vi "Get and Format debug data.vi"(7 "Table Control refnum":refnum<vi>, 9 "Update table position?":bool=TRUE, 10 "Format debug data?":bool, 11 "Empty debug data?":bool) -> (2 "Formatted debug data":string, 3 "Debug data array":T1[](array[typedef]) {"Time Stamp" format="%<%.3X %x>T"})   [LabVIEW 2019, in "ACSVcontrol-driver.lvlib"]
doc: "If debug mode was set on (use Initialize Globals), VI returns debug data.\nClears debug data if set.\nReturns debug data formatted as tab separated text if set.\nIf Table refnum exist, adds debug data into table. If set, the last shown row of the table is moved to show last row.\n\nDebug data are:\n- Time stamp\n- Write or Read\n- Status of Labview error after writing/reading all data\n- Data (TCP/IP message)\n- Code of Labview error\n- Source of Labview error\n- Call chain"
uses:
  ACSVcontrol-driver.lvlib
  Private/Type definitions/Debug data.ctl
  Private/Globals.vi
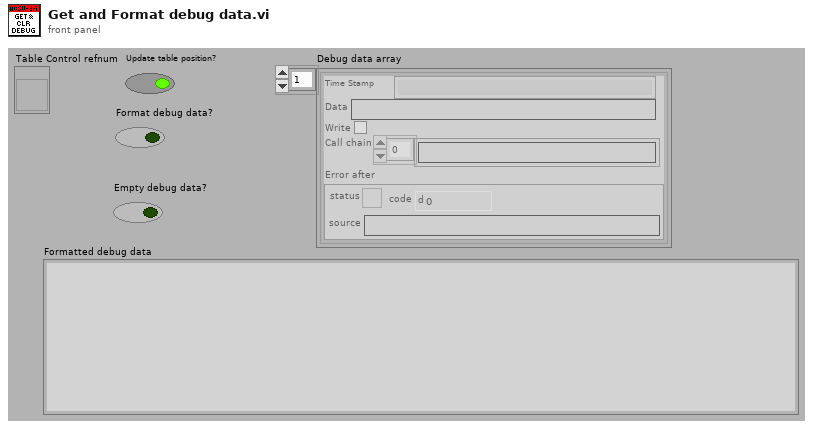
[diagram p1: front panel]
types:
  T1 = typedef "ACSVcontrol-driver.lvlib/Debug data.ctl" = cluster{"Time Stamp":timestamp, "Data":string, "Write":bool, "Call chain":string[], "Error after":errorcluster}
  T2 = typedef "LVRowAndColumnUnsignedTypeDef.ctl" = cluster{"Row":u32, "Column":u32}
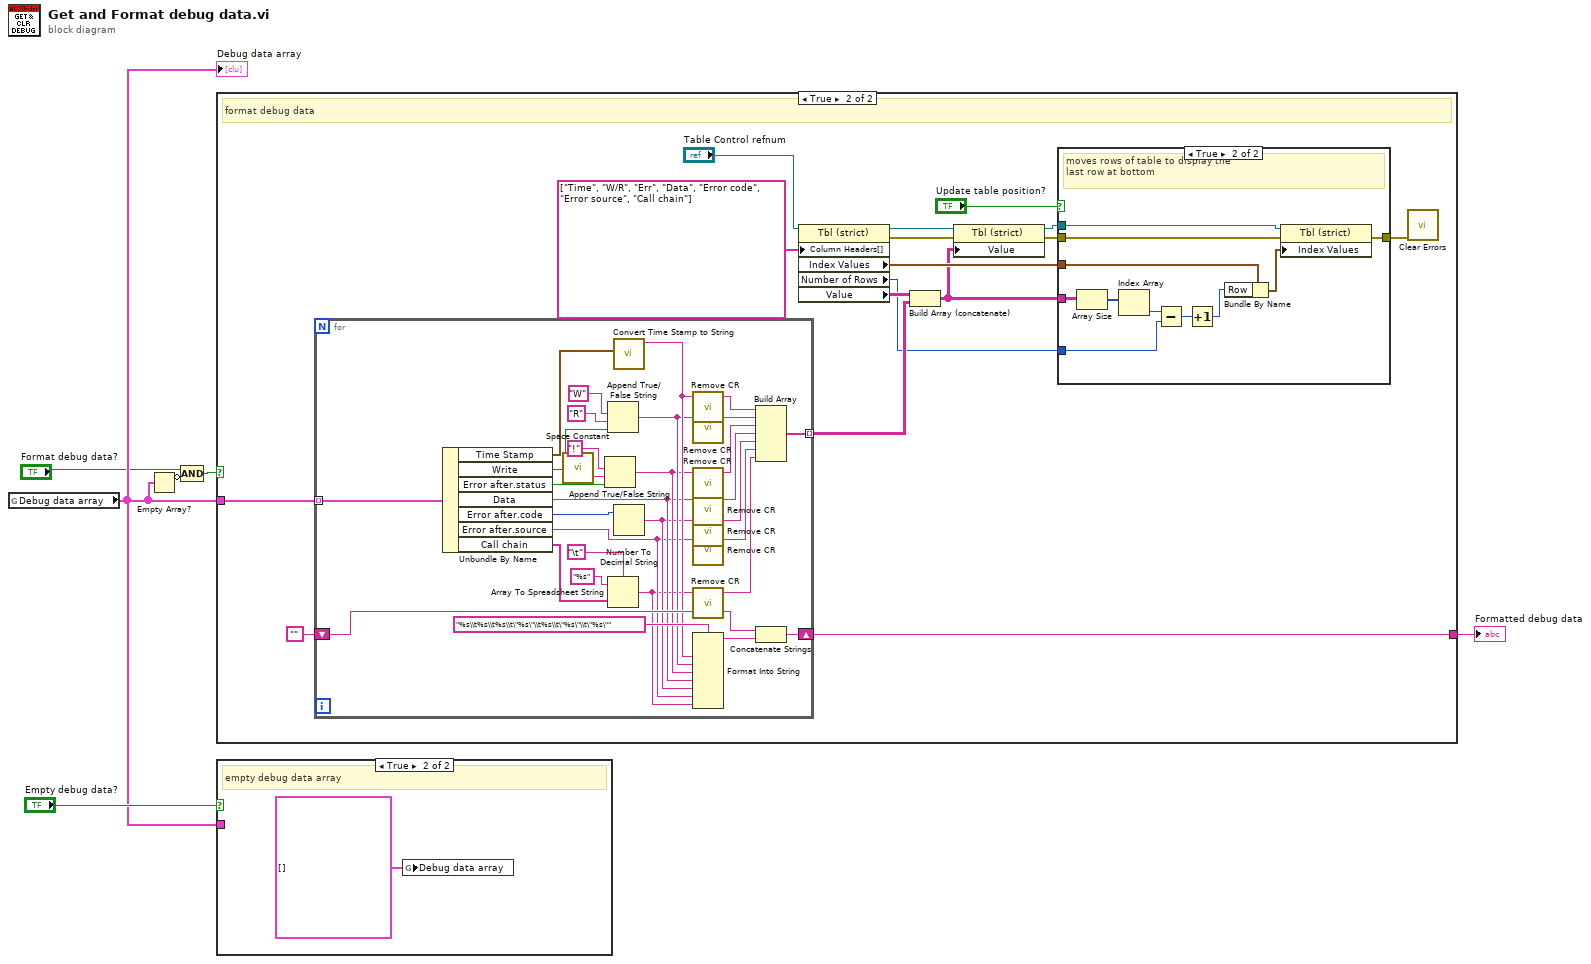
[diagram p0: block diagram]
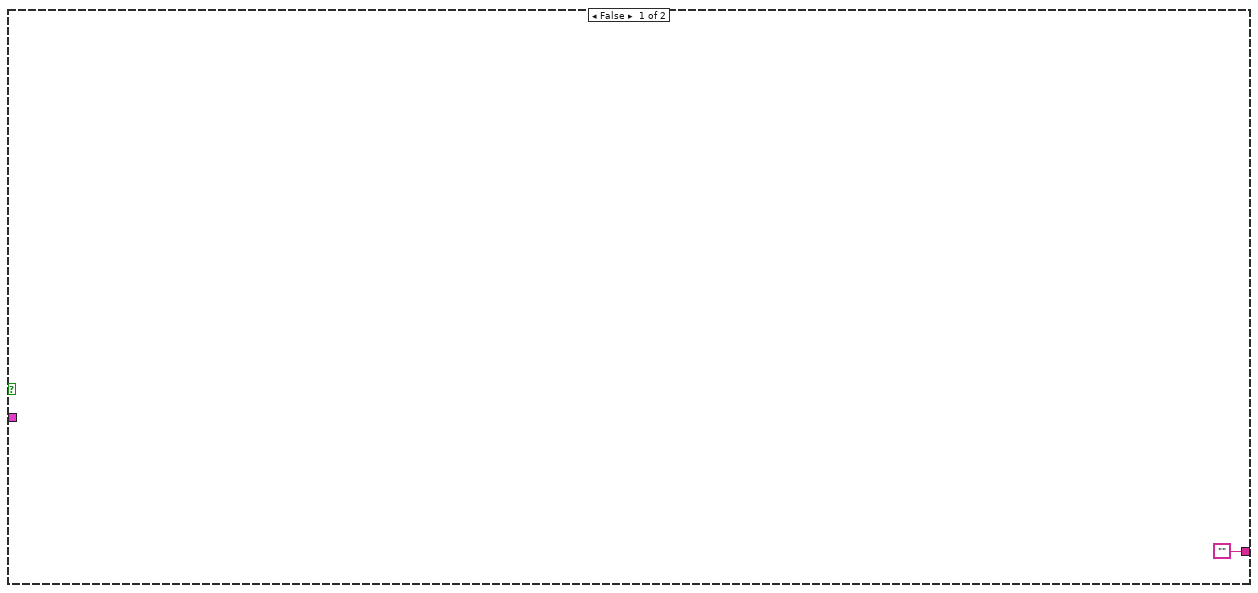
[diagram p2: hidden frame]
diagram:
  n1 = global read "Globals.vi" "Debug data array"() -> (w4:T1[])
  "Debug data array" <- w4
  n2 = Empty Array?(array=w4) -> (empty?=w3:bool)
  n3 = Compound Arithmetic op=AND("Format debug data?", invert w3) -> (w1:bool)
  n4 = case shown="True" w1 {
    tunnel: w4 -> [_ w23]
    tunnel: ["" w21] -> w5
    frame False {
    }
    frame True {
      # "format debug data"
      n5 = for {
        tunnel: w23 -> [w66] mode=indexing
        shift-right: [w54] -> w21
        shift-left: "" -> [w55]
        tunnel: [w53] -> w20 mode=indexing
        n6 = Unbundle By Name(w66) -> ("Time Stamp"=w65:timestamp, "Write"=w61:bool, "Error after.status"=w50:bool, "Data"=w46:string, "Error after.code"=w51:i32, "Error after.source"=w44:string, "Call chain"=w52:string[])
        n7 = call <vilib>:"Space Constant.vi"() -> ("String"=w59:string)
        n8 = Append True/False String(1:w50, 2:w59, 3:"!" ("true string")) -> (0:w47:string)  [unwired: 1 in]
        n9 = Append True/False String(1:w61, 2:"R" ("false string"), 3:"W" ("true string")) -> (0:w48:string)  [unwired: 1 in]
        n10 = Array To Spreadsheet String(delimiter (Tab)="\t", array=w52, 3:"%s" ("format string")) -> (spreadsheet string=w43:string)
        n11 = call "Convert Time Stamp to String.vi"("time stamp"=w65) -> ("date/time string"=w49:string)  [unwired: 10 in]
        n12 = Number To Decimal String(number=w51) -> (decimal integer string=w45:string)  [unwired: 1 in]
        n13 = call "Remove CR.vi"("string"=w49) -> ("string out"=w36:string)  [unwired: 4 in]
        n14 = call "Remove CR.vi"("string"=w48) -> ("string out"=w37:string)  [unwired: 4 in]
        n15 = call "Remove CR.vi"("string"=w47) -> ("string out"=w38:string)  [unwired: 4 in]
        n16 = call "Remove CR.vi"("string"=w46) -> ("string out"=w39:string)  [unwired: 4 in]
        n17 = call "Remove CR.vi"("string"=w45) -> ("string out"=w40:string)  [unwired: 4 in]
        n18 = call "Remove CR.vi"("string"=w44) -> ("string out"=w41:string)  [unwired: 4 in]
        n19 = call "Remove CR.vi"("string"=w43) -> ("string out"=w42:string)  [unwired: 4 in]
        n20 = Format Into String(format string="%s\\t%s\\t%s\\t\"%s\"\\t%s\\t\"%s\"\\t\"%s\"", w49, w48, w47, w46, w45, w44, w43) -> (resulting string=w56:string)  [unwired: 2 in, 1 out]
        n21 = Build Array(w36, w37, w38, w39, w40, w41, w42) -> (w53:string[])
        n22 = Concatenate Strings(w55, w56) -> (w54:string)
      }
      n23 = property class="Tbl (strict)"(reference="Table Control refnum", "Column Headers[]"=string[] ["Time", "W/R", "Err", "Data", "Error code", "Error source", "Call chain"] ("appended array")) -> (reference out=w16:refnum<vi>, error out=w15:errorcluster, "Index Values"=w18:T2, "Number of Rows"=w13:u32, "Value"=w19:string[][])  [unwired: 1 in]
      n24 = Build Array (concatenate)(w19, w20) -> (w12:string[][])
      n25 = property class="Tbl (strict)"(reference=w16, error in=w15, "Value"=w12) -> (reference out=w17:refnum<vi>, error out=w14:errorcluster)
      n26 = case shown="True" "Update table position?" {
        tunnel: w18 -> [_ w35]
        tunnel: w17 -> [_ w33]
        tunnel: w14 -> [w24 w32]
        tunnel: w13 -> [_ w31]
        tunnel: w12 -> [_ w30]
        tunnel: [w24 w25] -> w9
        frame False {
        }
        frame True {
          # "moves rows of table to display the\nlast row at bottom"
          n27 = Array Size(array=w30) -> (size(s)=w29:i32[])
          n28 = Index Array(array=w29) -> (element=w28:i32)  [unwired: 1 in]
          n29 = Subtract(x=w28, y=w31) -> (x-y=w27:u32)
          n30 = Increment(x=w27) -> (x+1=w26:u32)
          n31 = Bundle By Name(cluster=w35, "Row"=w26) -> (w34:T2)
          n32 = property class="Tbl (strict)"(reference=w33, error in=w32, "Index Values"=w34) -> (error out=w25:errorcluster)  [unwired: 1 out]
        }
      }
      n33 = call <vilib>:"Clear Errors.vi"("error in (no error)"=w9) -> ()  [unwired: 5 in, 2 out]
    }
  }
  "Formatted debug data" <- w5
  n34 = case shown="True" "Empty debug data?" {
    tunnel: w4 -> [_ _]
    frame False {
    }
    frame True {
      # "empty debug data array"
      n35 = global write "Globals.vi" "Debug data array"(T1[] [] ("Debug data array")) -> ()
    }
  }
